vi "Valve_Control.vi"() -> ()   [LabVIEW 2018]
uses:
  <vilib>/DAQmx/write.llb/DAQmx Write (Digital 1D Bool NChan 1Samp 1Line).vi
  <vilib>/DAQmx/create/channels.llb/DAQmx Create Channel (DO-Digital Output).vi
  <vilib>/Utility/file.llb/Read Delimited Spreadsheet (DBL).vi
  <vilib>/DAQmx/miscellaneous.llb/DAQmx Fill In Error Info.vi
panel:
  in  "stop (T) 7":bool=TRUE caption="stop (T)"
  in  "stop (T) 5":bool=TRUE caption="stop (T)"
  in  "stop (T) 2":bool=TRUE caption="stop (T)"
  in  "stop (T) 3":bool=TRUE caption="stop (T)"
  in  "stop (T)":bool=TRUE
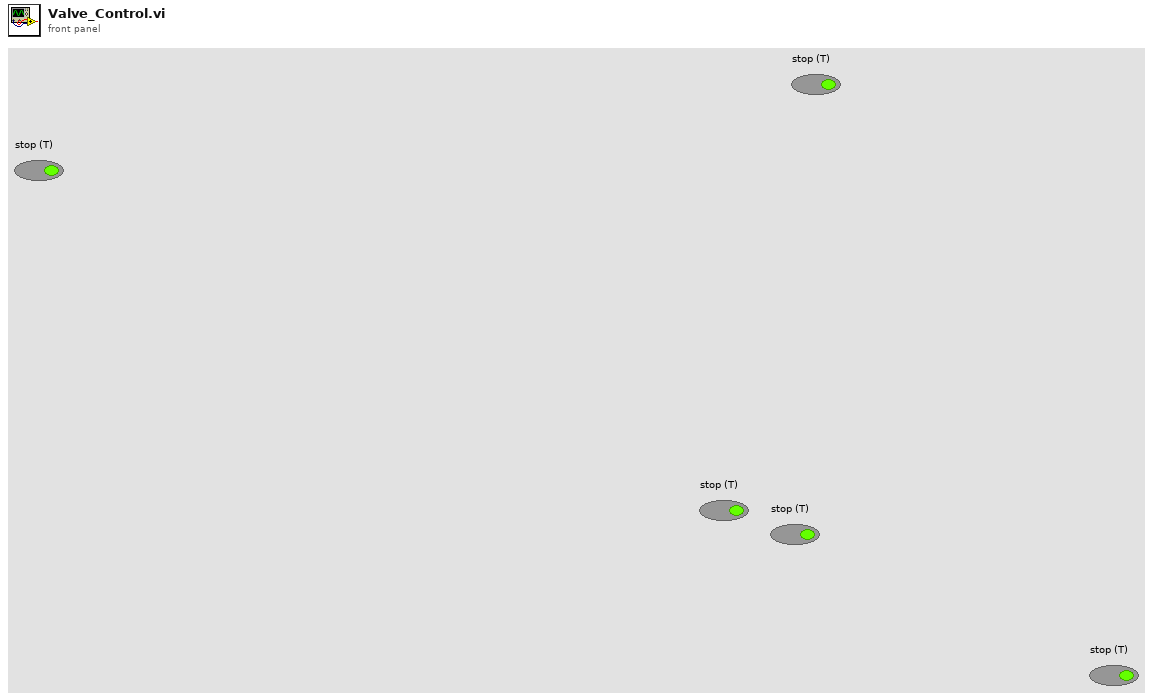
[diagram p1: front panel]
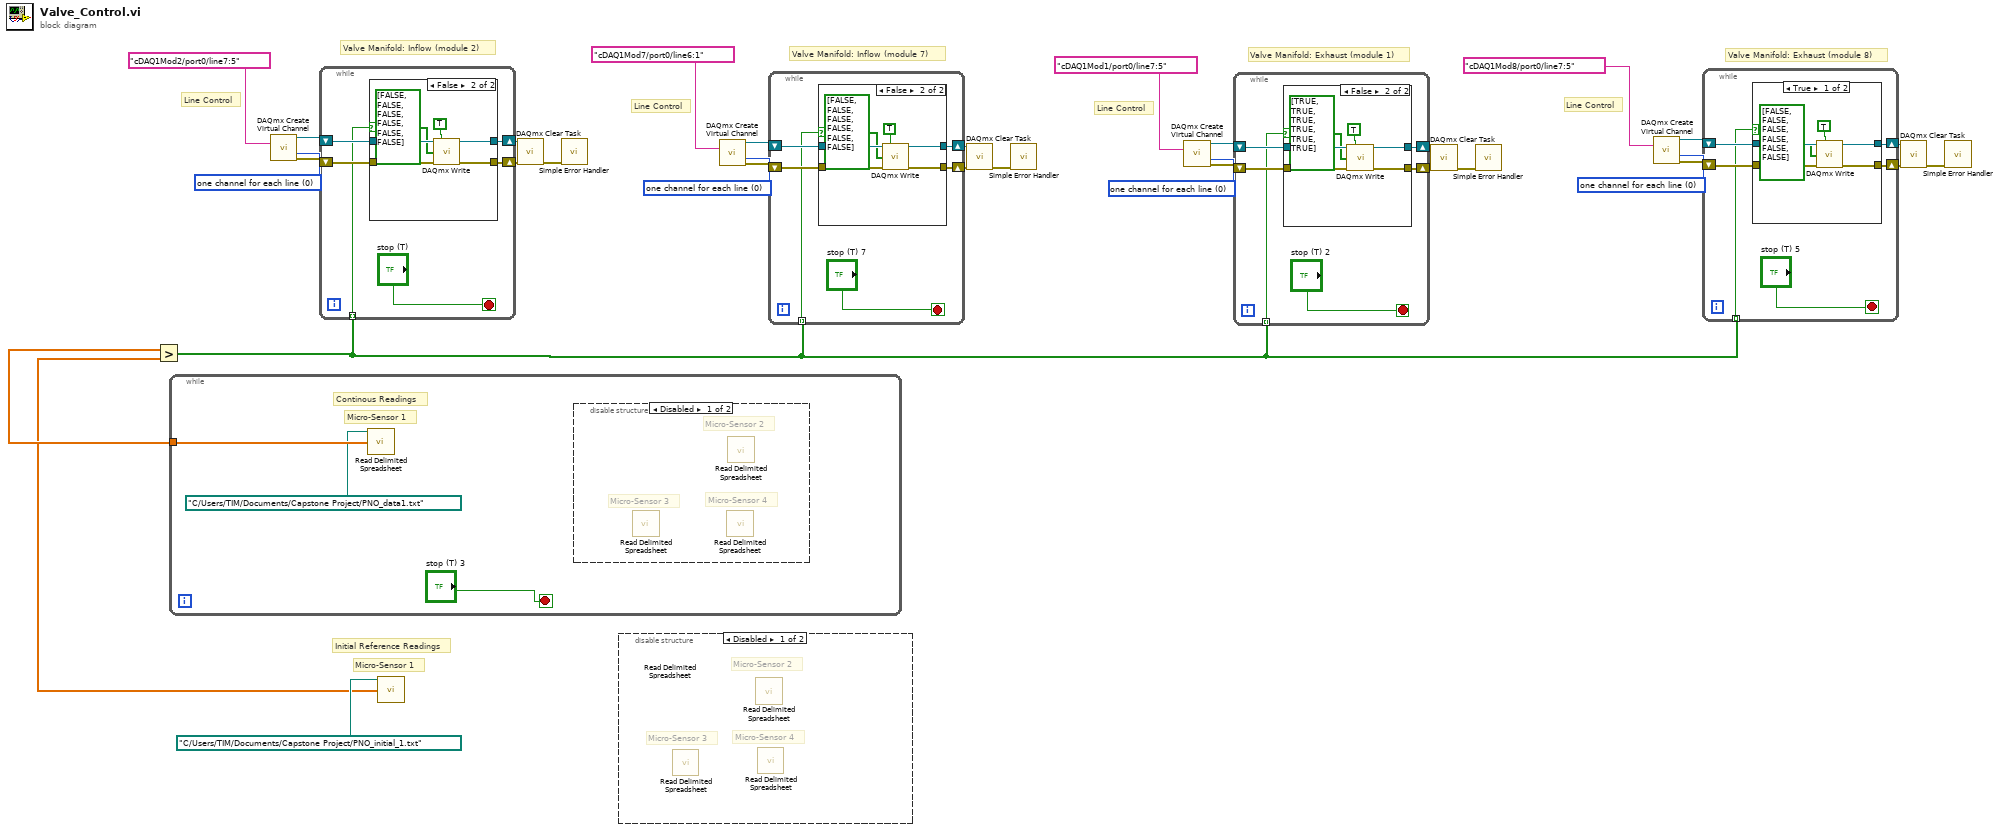
[diagram p0: block diagram]
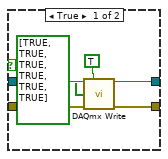
[diagram p2: hidden frame]
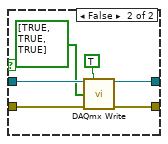
[diagram p3: hidden frame]
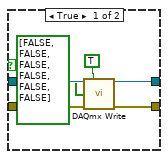
[diagram p4: hidden frame]
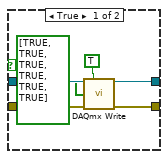
[diagram p7: hidden frame]
diagram:
  w2 = 0 items=["one channel for each line", "one channel for all lines"] ("line grouping")
  w9 = 0 items=["one channel for each line", "one channel for all lines"] ("line grouping")
  w16 = 0 items=["one channel for each line", "one channel for all lines"] ("line grouping")
  w26 = 0 items=["one channel for each line", "one channel for all lines"] ("line grouping")
  # "Valve Manifold: Inflow (module 7)"
  # "Line Control"
  # "Valve Manifold: Exhaust (module 8)"
  # "Valve Manifold: Exhaust (module 1)"
  # "Line Control"
  # "Line Control"
  # "Valve Manifold: Inflow (module 2)"
  # "Micro-Sensor 1"
  # "Initial Reference Readings"
  # "Line Control"
  n1 = while {
    tunnel: [w34] -> w24
    stop <- "stop (T) 3" stop-if-true
    # "Continous Readings"
    # "Micro-Sensor 1"
    n2 = call-poly <vilib>:"Read Delimited Spreadsheet.vi"("file path (dialog if empty)"=path "C:/Users/TIM/Documents/Capstone Project/PNO_data1.txt") -> ("first row"=w34:dbl[])  [unwired: 9 in, 5 out]
    n3 = disable-structure shown="Disabled" {
      frame Disabled {
        # "Micro-Sensor 4"
        # "Micro-Sensor 3"
        # "Micro-Sensor 2"
        n4 = call-poly <vilib>:"Read Delimited Spreadsheet.vi"() -> ()  [unwired: 10 in, 6 out]
        n5 = call-poly <vilib>:"Read Delimited Spreadsheet.vi"() -> ()  [unwired: 10 in, 6 out]
        n6 = call-poly <vilib>:"Read Delimited Spreadsheet.vi"() -> ()  [unwired: 10 in, 6 out]
      }
      frame Enabled {
      }
    }
  }
  n7 = call-poly <vilib>:"DAQmx Create Virtual Channel.vi"("lines"=tag "cDAQ1Mod2/port0/line7:5", "line grouping"=w26) -> ("task out"=w31:refnum<k21>, "error out"=w30:errorcluster)  [unwired: 12 in]
  n8 = call-poly <vilib>:"Read Delimited Spreadsheet.vi"("file path (dialog if empty)"=path "C:/Users/TIM/Documents/Capstone Project/PNO_initial_1.txt") -> ("first row"=w23:dbl[])  [unwired: 9 in, 5 out]
  n9 = Greater?(x=w24, y=w23) -> (0:w1:bool[])
  n10 = while {
    shift-right: [w39] -> w29
    shift-left: w31 -> [w41]
    shift-right: [w38] -> w28
    shift-left: w30 -> [w40]
    tunnel: w1 -> [w36] mode=indexing
    stop <- "stop (T)" stop-if-true
    n11 = case shown="False" w36 {
      tunnel: w41 -> [w47 w53]
      tunnel: w40 -> [w46 w52]
      tunnel: [w44 w50] -> w39
      tunnel: [w43 w49] -> w38
      frame True {
        n12 = call-poly <vilib>:"DAQmx Write.vi"("task/channels in"=w47, "auto start"=TRUE, "data"=bool[] [TRUE, TRUE, TRUE, TRUE, TRUE, TRUE], "error in"=w46) -> ("task out"=w44:refnum<k21>, "error out"=w43:errorcluster)  [unwired: 9 in, 1 out]
      }
      frame False {
        n13 = call-poly <vilib>:"DAQmx Write.vi"("task/channels in"=w53, "auto start"=TRUE, "data"=bool[] [FALSE, FALSE, FALSE, FALSE, FALSE, FALSE], "error in"=w52) -> ("task out"=w50:refnum<k21>, "error out"=w49:errorcluster)  [unwired: 9 in, 1 out]
      }
    }
  }
  n14 = call <vilib>:"DAQmx Clear Task.vi"("task in"=w29, "error in"=w28) -> ("error out"=w27:errorcluster)  [unwired: 13 in]
  n15 = call <vilib>:"Simple Error Handler.vi"("error in (no error)"=w27) -> ()  [unwired: 4 in, 5 out]
  n16 = disable-structure shown="Disabled" {
    frame Disabled {
      # "Micro-Sensor 4"
      # "Micro-Sensor 3"
      # "Micro-Sensor 2"
      n17 = call-poly <vilib>:"Read Delimited Spreadsheet.vi"() -> ()  [unwired: 10 in, 6 out]
      n18 = call-poly <vilib>:"Read Delimited Spreadsheet.vi"() -> ()  [unwired: 10 in, 6 out]
      n19 = call-poly <vilib>:"Read Delimited Spreadsheet.vi"() -> ()  [unwired: 10 in, 6 out]
    }
    frame Enabled {
    }
  }
  n20 = call-poly <vilib>:"DAQmx Create Virtual Channel.vi"("lines"=tag "cDAQ1Mod7/port0/line6:1", "line grouping"=w2) -> ("task out"=w7:refnum<k21>, "error out"=w6:errorcluster)  [unwired: 12 in]
  n21 = while {
    shift-right: [w57] -> w5
    shift-left: w7 -> [w59]
    shift-right: [w56] -> w4
    shift-left: w6 -> [w58]
    tunnel: w1 -> [w54] mode=indexing
    stop <- "stop (T) 7" stop-if-true
    n22 = case shown="False" w54 {
      tunnel: w59 -> [w65 w71]
      tunnel: w58 -> [w64 w70]
      tunnel: [w62 w68] -> w57
      tunnel: [w61 w67] -> w56
      frame True {
        n23 = call-poly <vilib>:"DAQmx Write.vi"("task/channels in"=w65, "auto start"=TRUE, "data"=bool[] [TRUE, TRUE, TRUE, TRUE, TRUE, TRUE], "error in"=w64) -> ("task out"=w62:refnum<k21>, "error out"=w61:errorcluster)  [unwired: 9 in, 1 out]
      }
      frame False {
        n24 = call-poly <vilib>:"DAQmx Write.vi"("task/channels in"=w71, "auto start"=TRUE, "data"=bool[] [FALSE, FALSE, FALSE, FALSE, FALSE, FALSE], "error in"=w70) -> ("task out"=w68:refnum<k21>, "error out"=w67:errorcluster)  [unwired: 9 in, 1 out]
      }
    }
  }
  n25 = call <vilib>:"DAQmx Clear Task.vi"("task in"=w5, "error in"=w4) -> ("error out"=w3:errorcluster)  [unwired: 13 in]
  n26 = call <vilib>:"Simple Error Handler.vi"("error in (no error)"=w3) -> ()  [unwired: 4 in, 5 out]
  n27 = call-poly <vilib>:"DAQmx Create Virtual Channel.vi"("lines"=tag "cDAQ1Mod1/port0/line7:5", "line grouping"=w16) -> ("task out"=w21:refnum<k21>, "error out"=w20:errorcluster)  [unwired: 12 in]
  n28 = while {
    shift-right: [w75] -> w19
    shift-left: w21 -> [w77]
    shift-right: [w74] -> w18
    shift-left: w20 -> [w76]
    tunnel: w1 -> [w72] mode=indexing
    stop <- "stop (T) 2" stop-if-true
    n29 = case shown="False" w72 {
      tunnel: w77 -> [w83 w89]
      tunnel: w76 -> [w82 w88]
      tunnel: [w80 w86] -> w75
      tunnel: [w79 w85] -> w74
      frame True {
        n30 = call-poly <vilib>:"DAQmx Write.vi"("task/channels in"=w83, "auto start"=TRUE, "data"=bool[] [FALSE, FALSE, FALSE, FALSE, FALSE, FALSE], "error in"=w82) -> ("task out"=w80:refnum<k21>, "error out"=w79:errorcluster)  [unwired: 9 in, 1 out]
      }
      frame False {
        n31 = call-poly <vilib>:"DAQmx Write.vi"("task/channels in"=w89, "auto start"=TRUE, "data"=bool[] [TRUE, TRUE, TRUE, TRUE, TRUE, TRUE], "error in"=w88) -> ("task out"=w86:refnum<k21>, "error out"=w85:errorcluster)  [unwired: 9 in, 1 out]
      }
    }
  }
  n32 = call <vilib>:"DAQmx Clear Task.vi"("task in"=w19, "error in"=w18) -> ("error out"=w17:errorcluster)  [unwired: 13 in]
  n33 = call <vilib>:"Simple Error Handler.vi"("error in (no error)"=w17) -> ()  [unwired: 4 in, 5 out]
  n34 = call-poly <vilib>:"DAQmx Create Virtual Channel.vi"("lines"=tag "cDAQ1Mod8/port0/line7:5", "line grouping"=w9) -> ("task out"=w14:refnum<k21>, "error out"=w13:errorcluster)  [unwired: 12 in]
  n35 = while {
    shift-right: [w93] -> w12
    shift-left: w14 -> [w95]
    shift-right: [w92] -> w11
    shift-left: w13 -> [w94]
    tunnel: w1 -> [w90] mode=indexing
    stop <- "stop (T) 5" stop-if-true
    n36 = case shown="True" w90 {
      tunnel: w95 -> [w101 w107]
      tunnel: w94 -> [w100 w106]
      tunnel: [w98 w104] -> w93
      tunnel: [w97 w103] -> w92
      frame True {
        n37 = call-poly <vilib>:"DAQmx Write.vi"("task/channels in"=w101, "auto start"=TRUE, "data"=bool[] [FALSE, FALSE, FALSE, FALSE, FALSE, FALSE], "error in"=w100) -> ("task out"=w98:refnum<k21>, "error out"=w97:errorcluster)  [unwired: 9 in, 1 out]
      }
      frame False {
        n38 = call-poly <vilib>:"DAQmx Write.vi"("task/channels in"=w107, "auto start"=TRUE, "data"=bool[] [TRUE, TRUE, TRUE], "error in"=w106) -> ("task out"=w104:refnum<k21>, "error out"=w103:errorcluster)  [unwired: 9 in, 1 out]
      }
    }
  }
  n39 = call <vilib>:"DAQmx Clear Task.vi"("task in"=w12, "error in"=w11) -> ("error out"=w10:errorcluster)  [unwired: 13 in]
  n40 = call <vilib>:"Simple Error Handler.vi"("error in (no error)"=w10) -> ()  [unwired: 4 in, 5 out]
